vi "Disconnect.vi"(8 "error in":errorcluster, 11 "6509 in":refnum<class "6509.lvclass">) -> (0 "error out":errorcluster, 3 "6509 out":refnum<class "6509.lvclass">)   [LabVIEW 2019, in "6509.lvlib" / "6509.lvclass"]
uses:
  Library/6509.lvclass
  C:/Users/Public/Documents/Development/builds/Instruments/DIG_IO.lvlibp/Library/DIG_IO.lvclass
  Library/6509.lvclass/6509.ctl
  builds/Instruments/DIG_IO.lvlibp/Accessors/Read IO_Mode.vi
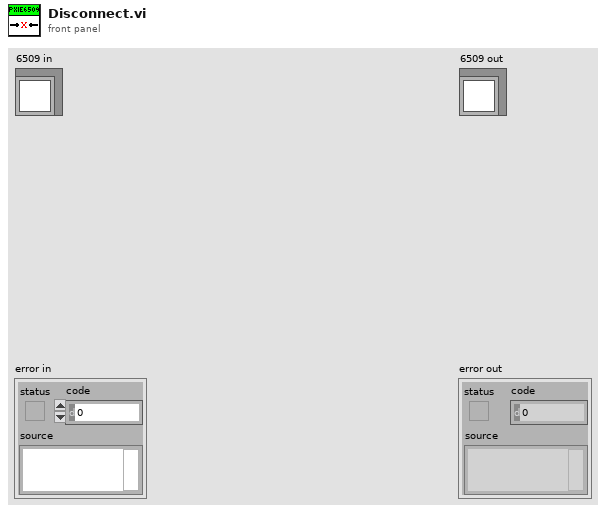
[diagram p1: front panel]
types:
  T1 = typedef "DIG_IO.lvlibp/DIG_IO.lvclass/IO Mode.ctl" = enum16{"IO", "IN", "OUT"}
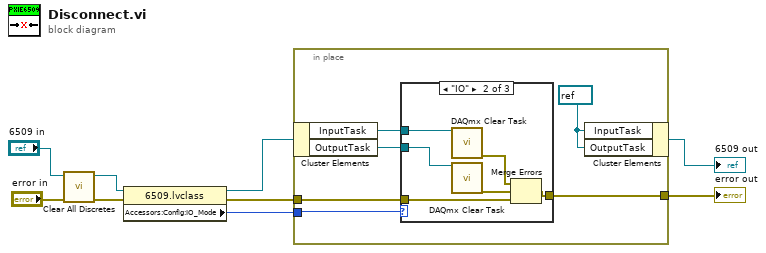
[diagram p0: block diagram]
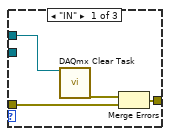
[diagram p2: hidden frame]
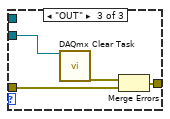
[diagram p3: hidden frame]
diagram:
  n1 = call-dynamic "Clear All Discretes.vi"("error in"="error in", "6509 in"="6509 in") -> ("error out"=w5:errorcluster, "6509 out"=w3:refnum<class "6509.lvclass">)  [unwired: 8 in]
  n2 = property class="6509.lvclass"(reference=w3, error in=w5) -> (reference out=w2:refnum<class "6509.lvclass">, error out=w4:errorcluster, "Accessors:Config:IO_Mode"=w1:T1)
  n3 = in-place {
    in-place-border: [w15] -> w9
    in-place-border: w4 -> [w14]
    in-place-border: w1 -> [w10]
    w13 = refnum<k21> refnum ("Local Resource")
    n4 = in-place-cluster #1(w2) -> ("InputTask"=w12:refnum<k21>, "OutputTask"=w11:refnum<k21>)
    n5 = case shown="\"IO\"" w10 {
      tunnel: [w19 w25 w29] -> w15
      tunnel: w14 -> [w17 w23 w27]
      tunnel: w12 -> [w16 w21 _]
      tunnel: w11 -> [_ w22 w26]
      frame "IN" {
        n6 = call <vilib>:"DAQmx Clear Task.vi"("task in"=w16) -> ("error out"=w18:errorcluster)  [unwired: 14 in]
        n7 = Merge Errors(w18, w17) -> (w19:errorcluster)
      }
      frame "IO" {
        n8 = call <vilib>:"DAQmx Clear Task.vi"("task in"=w21) -> ("error out"=w20:errorcluster)  [unwired: 14 in]
        n9 = call <vilib>:"DAQmx Clear Task.vi"("task in"=w22) -> ("error out"=w24:errorcluster)  [unwired: 14 in]
        n10 = Merge Errors(w20, w24, w23) -> (w25:errorcluster)
      }
      frame "OUT" {
        n11 = call <vilib>:"DAQmx Clear Task.vi"("task in"=w26) -> ("error out"=w28:errorcluster)  [unwired: 14 in]
        n12 = Merge Errors(w28, w27) -> (w29:errorcluster)
      }
    }
    n13 = in-place-cluster #1("InputTask"=w13, "OutputTask"=w13) -> (→"6509 out":refnum<class "6509.lvclass">)
  }
  "error out" <- w9
